vi "Kinect Open Baseline Image.vi"(8 "error in (no error)":errorcluster) -> (0 "error out":errorcluster, 2 "dup path":path, 3 "Image Out":T1)   [LabVIEW 2011]
uses:
  <vilib>/vision/Image Controls.llb/IMAQ Image.ctl
  <vilib>/Utility/sysdir.llb/System Directory Type.ctl
  Kinect Global Status.vi
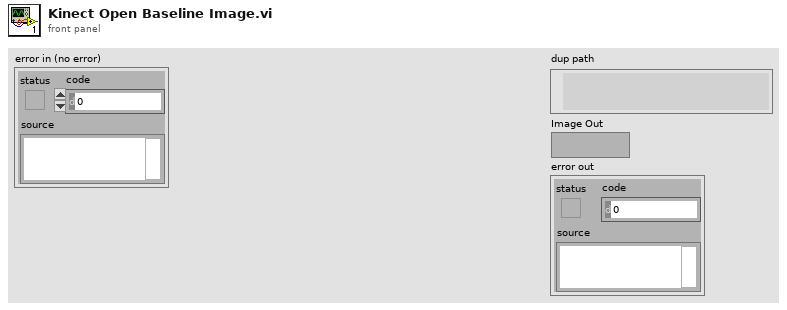
[diagram p1: front panel]
types:
  T1 = typedef "IMAQ Image.ctl" = refnum<image>
  T2 = typedef "System Directory Type.ctl" = i32
  T3 = typedef "Image Type" = u32
  T4 = cluster{"Image Height":i32, "Image Width":i32, "Minimum Framerate":i32, "Maximum Framerate":i32, "Framerate":i32, "Near Mode":bool, "Range":sgl}
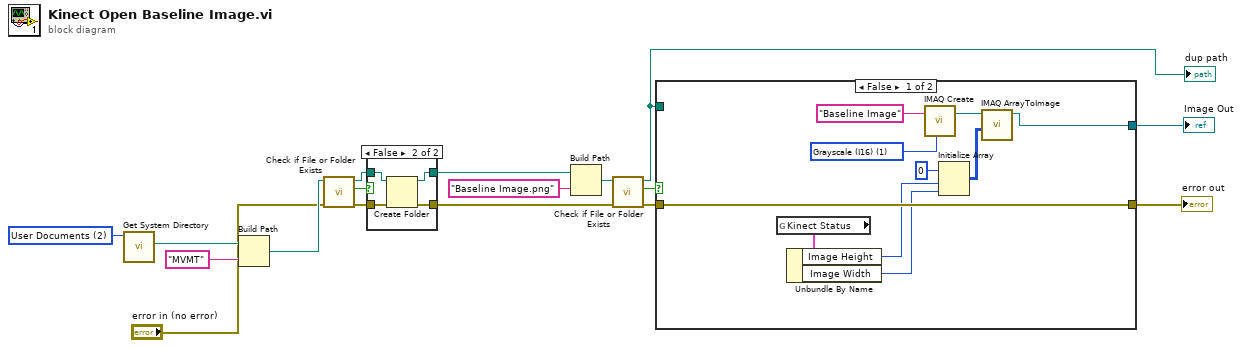
[diagram p0: block diagram]
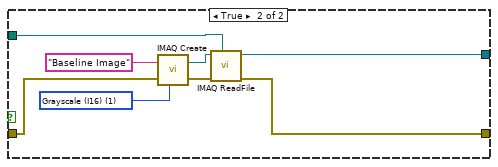
[diagram p2: hidden frame]
diagram:
  w6 = T2 2 items=["User Home"=0, "User Desktop"=1, "User Documents"=2, "User Application Data"=3, "User Preferences"=4, "User Temporary"=5, "Public Documents"=6, "Public Application Data"=7, "Public Preferences"=8, "Public Cache"=13, "System Core Libraries"=9, "System Installed Libraries"=10, "Application Files"=11, "Boot Volume Root"=12] ("system directory type")
  n1 = call <vilib>:"Get System Directory.vi"("system directory type"=w6) -> ("system directory"=w5:path)  [unwired: 10 in]
  n2 = Build Path(base path=w5, name or relative path="MVMT") -> (appended path=w14:path)
  n3 = call <vilib>:"Check if File or Folder Exists.vi"("error in (no error)"="error in (no error)", "path"=w14) -> ("error out"=w15:errorcluster, "file or folder exists?"=w17:bool, "dup path"=w16:path)  [unwired: 7 in]
  n4 = case shown="False" w17 {
    tunnel: w16 -> [w18 w23]
    tunnel: w15 -> [w19 w22]
    tunnel: [w18 w21] -> w12
    tunnel: [w19 w20] -> w9
    frame True {
    }
    frame False {
      n5 = Create Folder(path (use dialog)=w23, error in=w22) -> (created path=w21:path, error out=w20:errorcluster)  [unwired: 1 in, 1 out]
    }
  }
  n6 = Build Path(base path=w12, name or relative path="Baseline Image.png") -> (appended path=w10:path)
  n7 = call <vilib>:"Check if File or Folder Exists.vi"("error in (no error)"=w9, "path"=w10) -> ("error out"=w7:errorcluster, "file or folder exists?"=w8:bool, "dup path"=w4:path)  [unwired: 7 in]
  "dup path" <- w4
  n8 = case shown="False" w8 {
    tunnel: w7 -> [w33 w36]
    tunnel: [w33 w35] -> w2
    tunnel: [w27 w34] -> w3
    tunnel: w4 -> [_ w41]
    frame False {
      w29 = T3 1 items=["Grayscale (U8)", "Grayscale (I16)", "Grayscale (SGL)", "Complex (CSG)", "RGB (U32)", "HSL (U32)", "RGB (U64)", "Grayscale (U16)"] ("Image Type")
      n9 = global read "Kinect Global Status.vi" "Kinect Status"() -> (w26:T4)
      n10 = Unbundle By Name(w26) -> ("Image Height"=w25:i32, "Image Width"=w24:i32)
      n11 = call "IMAQ Create"("Image Name"="Baseline Image", "Image Type"=w29) -> ("New Image"=w30:T1)  [unwired: 3 in, 1 out]
      n12 = Initialize Array(i16 0, w25, w24) -> (w31:i16[][])
      n13 = call "IMAQ ArrayToImage"("Image Pixels (I16)"=w31, "Image"=w30) -> ("Image Out"=w27:T1)  [unwired: 8 in, 1 out]
    }
    frame True {
      w37 = T3 1 items=["Grayscale (U8)", "Grayscale (I16)", "Grayscale (SGL)", "Complex (CSG)", "RGB (U32)", "HSL (U32)", "RGB (U64)", "Grayscale (U16)"] ("Image Type")
      n14 = call "IMAQ Create"("Image Name"="Baseline Image", "Image Type"=w37, "error in (no error)"=w36) -> ("New Image"=w40:T1, "error out"=w39:errorcluster)  [unwired: 2 in]
      n15 = call "IMAQ ReadFile"("File Path"=w41, "error in (no error)"=w39, "Image"=w40) -> ("error out"=w35:errorcluster, "Image Out"=w34:T1)  [unwired: 4 in, 3 out]
    }
  }
  "Image Out" <- w3
  "error out" <- w2
